vi "instance count allowed.vi"(8 "error in":errorcluster, 11 "CEF_Configuration in":refnum<class "CEF_serializable configuration.lvclass">) -> (0 "error out":errorcluster, 2 "instances allowed":i32, 3 "CEF_Configuration out":refnum<class "CEF_serializable configuration.lvclass">)   [LabVIEW 2023, in "CEF.lvlib" / "CEF_serializable configuration.lvclass"]
doc: "Provides an interface for determining the reentrancy of the runtime class associated with this configuration class. For example, a module which performs processing tasks may allow for unlimited instances (-1) while a component which implements a TCP server may want to limit itself to a smaller number in order to preserve ports. configuration.lvclass provides a value of 0, as no runtime class exists for this configuration.Copyright 2017 National Instruments Corporation\n\nLicensed under the Apache License, Version 2.0 (the \"License\"); you may not use this file except in compliance with the License. You may obtain a copy of the License at http://www.apache.org/licenses/LICENSE-2.0\nUnless required by applicable law or agreed to in writing, software distributed under the License is distributed on an \"AS IS\" BASIS, WITHOUT WARRANTIES OR CONDITIONS OF ANY KIND, either express or implied. See the License for the specific language governing permissions and limitations under the License."
uses:
  CEF_serializable configuration.lvclass
  CEF.lvlib
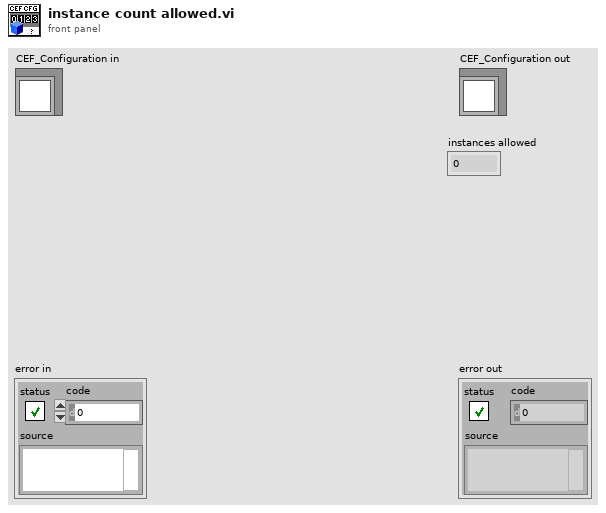
[diagram p1: front panel]
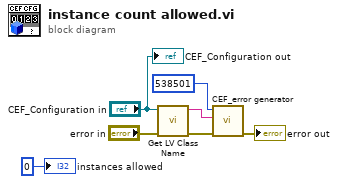
[diagram p0: block diagram]
diagram:
  n1 = call <vilib>:"Get LV Class Name.vi"("error in (no error)"="error in", "object"="CEF_Configuration in") -> ("error out"=w3:errorcluster, "class name"=w1:string)  [unwired: 8 in]
  n2 = call "CEF_error generator.vi"("error in"=w3, "append error message"=w1, "error code (0)"=538501) -> ("error out"=→"error out":errorcluster)  [unwired: 6 in]
  "CEF_Configuration out" <- "CEF_Configuration in"
  "instances allowed" <- 0 ("instances allowed (-1 = no limit)")
